vi "Autonomous Independent.vi"   [LabVIEW 2011]
doc: "This VI is called when autonomous begins, and will automatically be terminated when autonomous ends. You can carry out timed or sensor driven robot movement independently without needing to return to the caller."
uses:
  Robot Global Data.vi
types:
  T1 = typedef "WPI_DigitalInputDevRef.ctl" = cluster{"DevStatus":errorcluster, "DIO Channel":T2, "Digital Module":T3}
  T2 = typedef "FPGA_DIOChannel.ctl" = enum8{"DIO 1", "DIO 2", "DIO 3", "DIO 4", "DIO 5", "DIO 6", "DIO 7", "DIO 8", "DIO 9", "DIO 10", "DIO 11", "DIO 12", "DIO 13", "DIO 14", "Invalid"}
  T3 = typedef "FPGA_TypedefDigitalModule.ctl" = enum16{"Digital Module 1", "Digital Module 2"}
  T4 = typedef "WPI_MotorControlDeviceRef.ctl" = cluster{"DeviceStatus":errorcluster, "Type":enum16{"PWM", "CAN"}, "PWM":cluster{"Digital Module":T3, "PWM Channel":T5, "DeadBand":T6}, "CAN":cluster{"Device Number":u8, "Control Mode":T7, "Semaphore":T8, "Max Vout":dbl}, "Invert":bool, "TransformRef":T9, "InvTransformRef":T9}
  T5 = typedef "FPGA_DIOPWMChannel.ctl" = enum8{"PWM 1", "PWM 2", "PWM 3", "PWM 4", "PWM 5", "PWM 6", "PWM 7", "PWM 8", "PWM 9", "PWM 10", "Invalid"}
  T6 = typedef "WPI_PWMDeadband.ctl" = cluster{"Name":string, "maxPositivePwm":i32, "minPositivePwm":i32, "centerPwm":i32, "maxNegativePwm":i32, "minNegativePwm":i32, "angularRange":u16}
  T7 = typedef "WPI_CANJaguar_ControlMode.ctl" = enum8{"Percent VBus", "Current", "Speed", "Position", "Voltage"}
  T8 = typedef "Semaphore RefNum" = refnum<k1>
  T9 = typedef "WPI_PWMTransform_ConPane.ctl" = refnum<vi>
  T10 = typedef "WPI_JoystickDevRef.ctl" = cluster{"Device":T11}
  T11 = typedef "WPI_JoystickDeviceEnum.ctl" = enum16{"USB 1", "USB 2", "USB 3", "USB 4", "Kinect 1", "Kinect 2"}
  T12 = cluster{"axis 1 (x)":dbl, "axis 2 (y)":dbl, "axis 3 (throttle)":dbl, "axis 4":dbl, "axis 5":dbl, "axis 6":dbl}
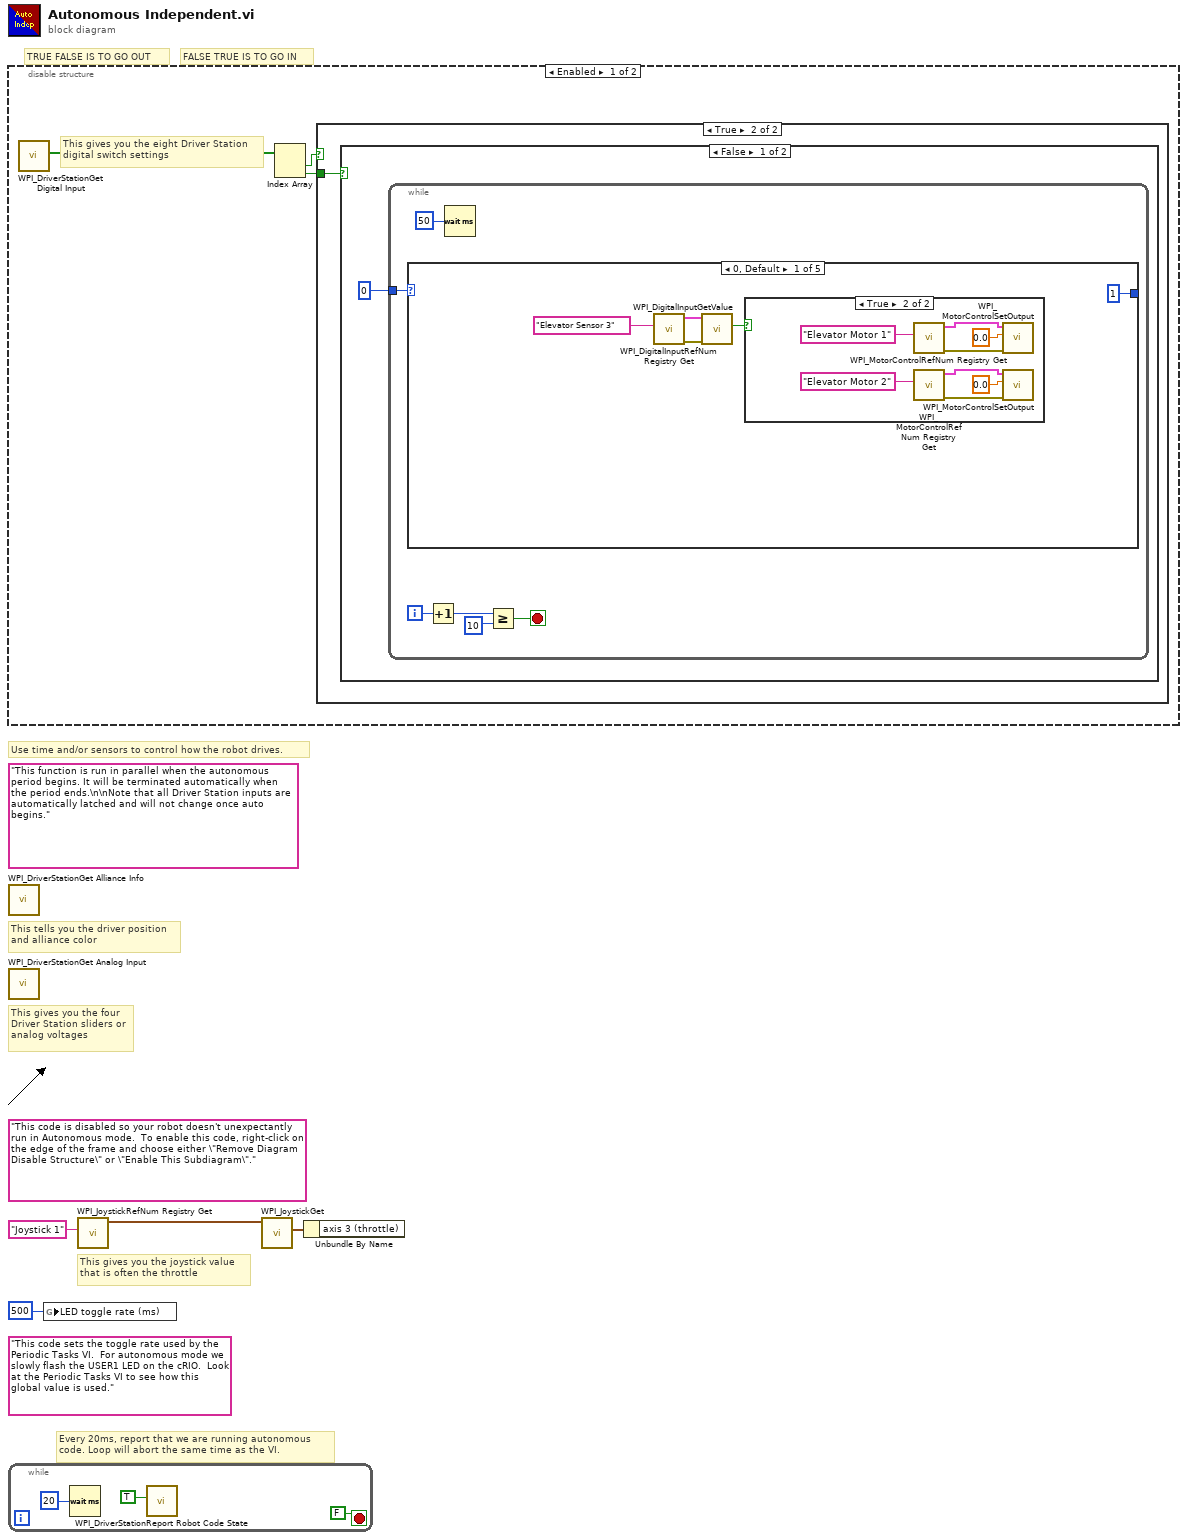
[diagram p0: block diagram]
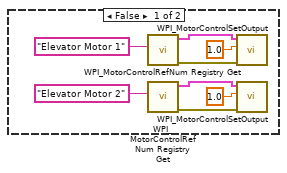
[diagram p4: hidden frame]
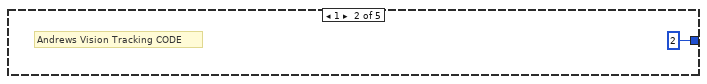
[diagram p5: hidden frame]
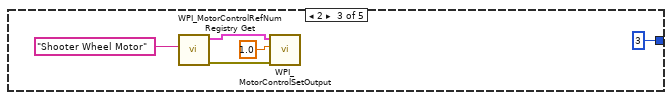
[diagram p6: hidden frame]
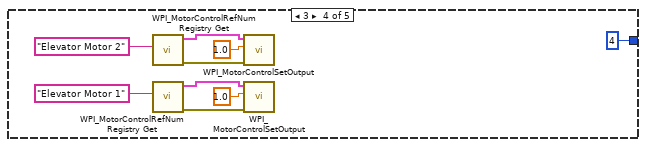
[diagram p7: hidden frame]
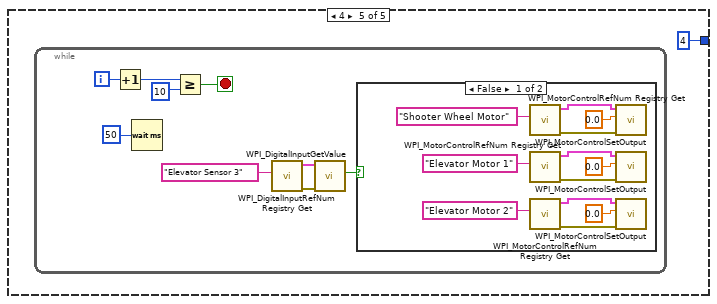
[diagram p8: hidden frame]
diagram:
  (unwired) "This code sets the toggle rate used by the Periodic Tasks VI.  For autonomous mode we slowly flash the USER1 LED on the cRIO.  Look at the Periodic Tasks VI to see how this global value is used."
  (unwired) "This code is disabled so your robot doesn't unexpectantly run in Autonomous mode.  To enable this code, right-click on the edge of the frame and choose either \"Remove Diagram Disable Structure\" or \"Enable This Subdiagram\"."
  (unwired) "This function is run in parallel when the autonomous period begins. It will be terminated automatically when the period ends.\n\nNote that all Driver Station inputs are automatically latched and will not change once auto begins."
  # "FALSE TRUE IS TO GO IN"
  # "TRUE FALSE IS TO GO OUT"
  # "Every 20ms, report that we are running autonomous\ncode. Loop will abort the same time as the VI."
  # "This gives you the joystick value\nthat is often the throttle"
  # "Use time and/or sensors to control how the robot drives."
  # "This tells you the driver position\nand alliance color"
  # "This gives you the four\nDriver Station sliders or\nanalog voltages"
  n1 = disable-structure shown="Enabled" {
    frame Enabled {
      # "This gives you the eight Driver Station\ndigital switch settings"
      n2 = call <vilib>:"WPI_DriverStationGet Digital Input.vi"() -> ("Driver Station Digital Input (1-8)"=w5:bool[])  [unwired: 11 out]
      n3 = Index Array(array=w5) -> (element #1=w6:bool, element #2=w7:bool)  [unwired: 2 in]
      n4 = case shown="True" w6 {
        tunnel: w7 -> [w8 w9]
        frame False {
          n5 = case shown="False" w8 {
            frame False {
            }
            frame True {
            }
          }
        }
        frame True {
          n6 = case shown="False" w9 {
            frame False {
              n7 = while {
                tunnel: 0 -> [w16]
                i -> [w11]
                stop <- w13 stop-if-true
                n8 = case shown="0, Default" w16 {
                  tunnel: [1 2 3 4 4] -> _
                  frame 0, Default {
                    n9 = call <vilib>:"WPI_DigitalInputRefNum Registry Get.vi"("refnum name"="Elevator Sensor 3") -> ("error out"=w21:errorcluster, "DigitalInputDevRef"=w20:T1)  [unwired: 9 in]
                    n10 = call <vilib>:"WPI_DigitalInputGetValue.vi"("error in (no error)"=w21, "DigitalInputDevRef"=w20) -> ("Value"=w18:bool)  [unwired: 7 in, 2 out]
                    n11 = case shown="True" w18 {
                      frame False {
                        n12 = call <vilib>:"WPI_MotorControlRefNum Registry Get.vi"("refnum name"="Elevator Motor 1") -> ("error out"=w26:errorcluster, "MotorControlDevRef"=w25:T4)  [unwired: 9 in]
                        n13 = call <vilib>:"WPI_MotorControlRefNum Registry Get.vi"("refnum name"="Elevator Motor 2") -> ("error out"=w29:errorcluster, "MotorControlDevRef"=w22:T4)  [unwired: 9 in]
                        n14 = call <vilib>:"WPI_MotorControlSetOutput.vi"("error in (no error)"=w26, "Output"=1.0, "MotorControlDevRef"=w25) -> ()  [unwired: 7 in, 2 out]
                        n15 = call <vilib>:"WPI_MotorControlSetOutput.vi"("error in (no error)"=w29, "Output"=1.0, "MotorControlDevRef"=w22) -> ()  [unwired: 7 in, 2 out]
                      }
                      frame True {
                        n16 = call <vilib>:"WPI_MotorControlRefNum Registry Get.vi"("refnum name"="Elevator Motor 1") -> ("error out"=w34:errorcluster, "MotorControlDevRef"=w33:T4)  [unwired: 9 in]
                        n17 = call <vilib>:"WPI_MotorControlRefNum Registry Get.vi"("refnum name"="Elevator Motor 2") -> ("error out"=w37:errorcluster, "MotorControlDevRef"=w30:T4)  [unwired: 9 in]
                        n18 = call <vilib>:"WPI_MotorControlSetOutput.vi"("error in (no error)"=w34, "Output"=0.0, "MotorControlDevRef"=w33) -> ()  [unwired: 7 in, 2 out]
                        n19 = call <vilib>:"WPI_MotorControlSetOutput.vi"("error in (no error)"=w37, "Output"=0.0, "MotorControlDevRef"=w30) -> ()  [unwired: 7 in, 2 out]
                      }
                    }
                  }
                  frame 1 {
                    # "Andrews Vision Tracking CODE"
                  }
                  frame 2 {
                    n20 = call <vilib>:"WPI_MotorControlRefNum Registry Get.vi"("refnum name"="Shooter Wheel Motor") -> ("error out"=w39:errorcluster, "MotorControlDevRef"=w42:T4)  [unwired: 9 in]
                    n21 = call <vilib>:"WPI_MotorControlSetOutput.vi"("error in (no error)"=w39, "Output"=1.0, "MotorControlDevRef"=w42) -> ()  [unwired: 7 in, 2 out]
                  }
                  frame 3 {
                    n22 = call <vilib>:"WPI_MotorControlRefNum Registry Get.vi"("refnum name"="Elevator Motor 2") -> ("error out"=w52:errorcluster, "MotorControlDevRef"=w51:T4)  [unwired: 9 in]
                    n23 = call <vilib>:"WPI_MotorControlRefNum Registry Get.vi"("refnum name"="Elevator Motor 1") -> ("error out"=w48:errorcluster, "MotorControlDevRef"=w47:T4)  [unwired: 9 in]
                    n24 = call <vilib>:"WPI_MotorControlSetOutput.vi"("error in (no error)"=w52, "Output"=1.0, "MotorControlDevRef"=w51) -> ()  [unwired: 7 in, 2 out]
                    n25 = call <vilib>:"WPI_MotorControlSetOutput.vi"("error in (no error)"=w48, "Output"=1.0, "MotorControlDevRef"=w47) -> ()  [unwired: 7 in, 2 out]
                  }
                  frame 4 {
                    n26 = while {
                      i -> [w54]
                      stop <- w56 stop-if-true
                      n27 = Increment(x=w54) -> (x+1=w57:i32)
                      n28 = Wait (ms)(milliseconds to wait=u32 50) -> ()  [unwired: 1 out]
                      n29 = Greater Or Equal?(x=w57, y=10) -> (x >= y?=w56:bool)
                      n30 = call <vilib>:"WPI_DigitalInputRefNum Registry Get.vi"("refnum name"="Elevator Sensor 3") -> ("error out"=w62:errorcluster, "DigitalInputDevRef"=w61:T1)  [unwired: 9 in]
                      n31 = call <vilib>:"WPI_DigitalInputGetValue.vi"("error in (no error)"=w62, "DigitalInputDevRef"=w61) -> ("Value"=w59:bool)  [unwired: 7 in, 2 out]
                      n32 = case shown="False" w59 {
                        frame False {
                          n33 = call <vilib>:"WPI_MotorControlRefNum Registry Get.vi"("refnum name"="Shooter Wheel Motor") -> ("error out"=w63:errorcluster, "MotorControlDevRef"=w66:T4)  [unwired: 9 in]
                          n34 = call <vilib>:"WPI_MotorControlRefNum Registry Get.vi"("refnum name"="Elevator Motor 1") -> ("error out"=w70:errorcluster, "MotorControlDevRef"=w69:T4)  [unwired: 9 in]
                          n35 = call <vilib>:"WPI_MotorControlRefNum Registry Get.vi"("refnum name"="Elevator Motor 2") -> ("error out"=w74:errorcluster, "MotorControlDevRef"=w73:T4)  [unwired: 9 in]
                          n36 = call <vilib>:"WPI_MotorControlSetOutput.vi"("error in (no error)"=w63, "Output"=0.0, "MotorControlDevRef"=w66) -> ()  [unwired: 7 in, 2 out]
                          n37 = call <vilib>:"WPI_MotorControlSetOutput.vi"("error in (no error)"=w70, "Output"=0.0, "MotorControlDevRef"=w69) -> ()  [unwired: 7 in, 2 out]
                          n38 = call <vilib>:"WPI_MotorControlSetOutput.vi"("error in (no error)"=w74, "Output"=0.0, "MotorControlDevRef"=w73) -> ()  [unwired: 7 in, 2 out]
                        }
                        frame True {
                        }
                      }
                    }
                  }
                }
                n39 = Increment(x=w11) -> (x+1=w14:i32)
                n40 = Wait (ms)(milliseconds to wait=u32 50) -> ()  [unwired: 1 out]
                n41 = Greater Or Equal?(x=w14, y=10) -> (x >= y?=w13:bool)
              }
            }
            frame True {
            }
          }
        }
      }
    }
    frame Disabled {
    }
  }
  n42 = call <vilib>:"WPI_DriverStationGet Alliance Info.vi"() -> ()  [unwired: 12 out]
  n43 = call <vilib>:"WPI_DriverStationGet Analog Input.vi"() -> ()  [unwired: 12 out]
  n44 = while {
    stop <- FALSE stop-if-true
    n45 = Wait (ms)(milliseconds to wait=u32 20) -> ()  [unwired: 1 out]
    n46 = call <vilib>:"WPI_DriverStationReport Robot Code State.vi"("Autonomous"=TRUE) -> ()  [unwired: 10 in, 1 out]
  }
  n47 = global write "Robot Global Data.vi" "LED toggle rate (ms)"(u32 500 ("LED ms toggle rate")) -> ()
  n48 = call <vilib>:"WPI_JoystickRefNum Registry Get.vi"("refnum name"="Joystick 1") -> ("JoystickDevRef"=w2:T10)  [unwired: 1 in, 9 out]
  n49 = call <vilib>:"WPI_JoystickGet.vi"("JoystickDevRef"=w2) -> ("Axes"=w3:T12)  [unwired: 1 in, 5 out]
  n50 = Unbundle By Name(w3) -> ()  [unwired: 1 out]
